vi "SeCrTS-DD AI V Search Channel.vi"(11 "AI Data":waveform(dbl)[](array[waveform])) -> (3 "FeedBack":dbl[](array[numeric]))   [LabVIEW 2022 SP3]
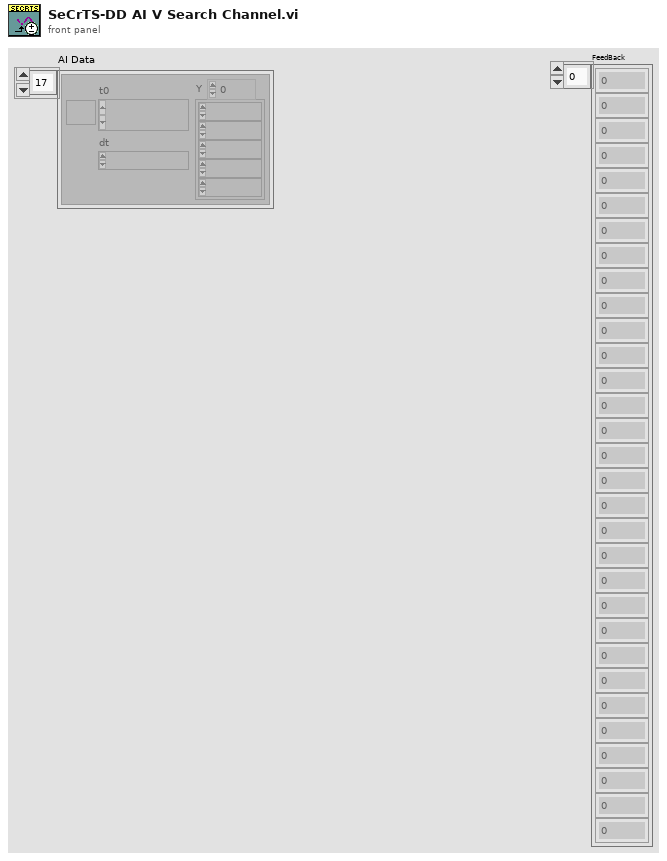
[diagram p1: front panel]
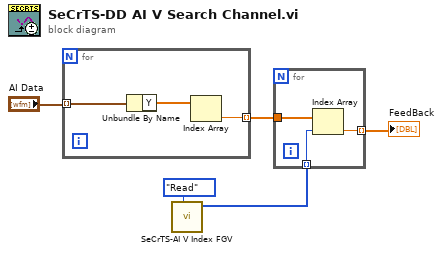
[diagram p0: block diagram]
diagram:
  n1 = for {
    tunnel: "AI Data" -> [w6] mode=indexing
    tunnel: [w7] -> w5 mode=indexing
    n2 = Unbundle By Name(w6) -> ("Y"=w8:dbl[])
    n3 = Index Array(array=w8) -> (element=w7:dbl)  [unwired: 1 in]
  }
  n4 = call "SeCrTS-AI V Index FGV .vi"("Action"=enum16{"Write", "Read", "Init"}."Read") -> ("Ai Index Element R"=w1:i32[])  [unwired: 10 in]
  n5 = for {
    tunnel: w5 -> [w11]
    tunnel: w1 -> [w10] mode=indexing
    tunnel: [w9] -> w4 mode=indexing
    n6 = Index Array(array=w11, index=w10) -> (element=w9:dbl)
  }
  "FeedBack" <- w4
